vi "Insert Named Instr.vi"(0 "new instrument":T1, 1 "Setup":T2[](array[typedef]) {"Private"."Offset" format="%^_3e"; "Private"."Scale Factors" format="%^_3e"}, 2 "Configured Names":string[](array[string]), 3 "Instrument List":i32) -> (5 "dup Setup":T2[](array[typedef]) {"Private"."Offset" format="%^_3e"; "Private"."Scale Factors" format="%^_3e"}, 7 "Item Names":string[](array[string]), 8 "Instrument List Out":i32)   [LabVIEW 2024]
uses:
  New NML Data Acq/Sub Controls/Instrument Properties.ctl
  New NML Data Acq/Sub Controls/Public.ctl
  New NML Data Acq/Sub Controls/Private.ctl
  New NML Data Acq/Sub Controls/Instrument Ref.ctl
  New NML Data Acq/Sub Controls/SystemCheckBox-resize.ctl
  Sub Controls/Instrument Info.ctl
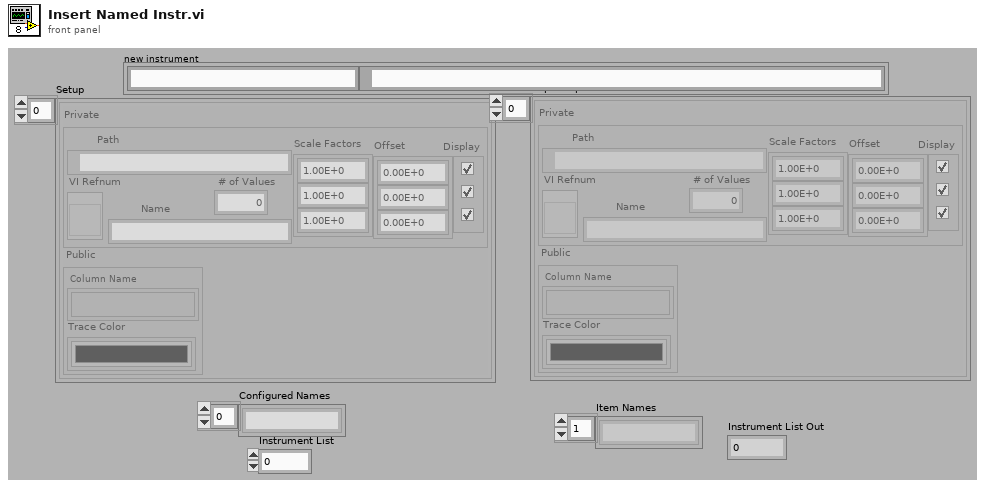
[diagram p1: front panel]
types:
  T1 = typedef "Instrument Info.ctl" = cluster{"Name":string, "path":path}
  T2 = typedef "Instrument Properties.ctl" = cluster{"Public":T3, "Private":T4}
  T3 = typedef "Public.ctl" = cluster{"Column Name":string[], "Trace Color":u32[]}
  T4 = typedef "Private.ctl" = cluster{"Path":path, "VI Refnum":T5, "Name":string, "# of Values":i32, "Scale Factors":dbl[], "Display":T6[], "Offset":dbl[]}
  T5 = typedef "Instrument Ref.ctl" = refnum<vi>
  T6 = typedef "SystemCheckBox-resize.ctl" = bool
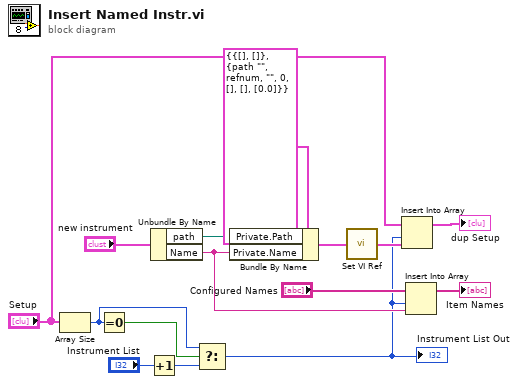
[diagram p0: block diagram]
diagram:
  n1 = Array Size(array="Setup") -> (size(s)=w1:i32)
  n2 = Equal To 0?(x=w1) -> (x = 0?=w2:bool)
  n3 = Increment(x="Instrument List") -> (x+1=w12:i32)
  n4 = Unbundle By Name("new instrument") -> ("path"=w6:path, "Name"=w5:string)
  n5 = Select(t=w1, s=w2, f=w12) -> (s? t:f=w4:i32)
  "Instrument List Out" <- w4
  n6 = Bundle By Name(cluster=T2 {"Public"={"Column Name"=[], "Trace Color"=[]}, "Private"={"Path"=path "", "VI Refnum"=refnum, "Name"="", "# of Values"=0, "Scale Factors"=[], "Display"=[], "Offset"=[0.0]}} ("Instrument Prop"), "Private.Path"=w6, "Private.Name"=w5) -> (w11:T2)
  n7 = call "Set VI Ref.vi"("Instrument Prop In"=w11) -> ("Instrument Prop Out"=w9:T2)
  n8 = Insert Into Array(array="Setup", index=w4, new element=w9) -> (→"dup Setup":T2[])
  n9 = Insert Into Array(array="Configured Names", index=w4, new element=w5) -> (→"Item Names":string[])
